vi "Live imaging-Generate images.vi"(4 "Left Channel":enum16{"Red Channel", "Green Channel"}(ring), 6 "Right Channel":enum16{"Red Channel", "Green Channel"}(ring), 10 "Images array":T1[](array[typedef]), 11 "Waveforms":waveform(dbl)[](array[waveform])) -> (0 "error out":errorcluster, 1 "Left image":T1, 3 "Right Image":T1)   [LabVIEW 2020]
uses:
  <vilib>/vision/Image Controls.llb/IMAQ Image.ctl
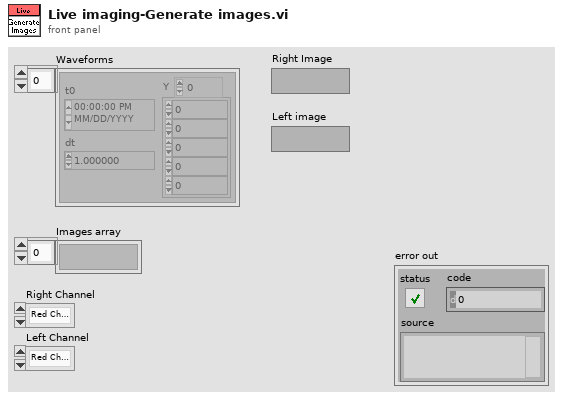
[diagram p1: front panel]
types:
  T1 = typedef "IMAQ Image.ctl" = refnum<image>
  T2 = typedef "AOL_Globals.ctl" = cluster{"Imaging Protocol":T3, "Number of POI":u16, "Number of Miniscans":u16, "Number of Trials":u16, "Number of Cycles ":u64, "# Averaged Frames":u16, "Laser power (%)":u8, "Pockels (V)":dbl, "Acquisition Length (sec)":dbl, "Fill time (us)":dbl, "POI Dwell time (us)":dbl, "Miniscan Dwell time per pixel (us)":dbl, "PMT 1":dbl, "PMT 2":dbl, "Back Apperture (mA)":dbl, "Frame Size":T4, "Center Frequency":dbl, "Field of View (norm)":dbl, "DwellTime (us)":dbl, "Wavelength (nm)":dbl, "Zoom":dbl, "AOL Z":dbl, "AOL Mode":T5, "GridXY":dbl, "GridZ":dbl, "TriggerPeriod (sec)":dbl, "Number of Pixels in Miniscan":u16, "Experiment folder path":path, "X centre":dbl, "Y centre":dbl, "Angle (degrees)":dbl, "Plane Mode":T6, "Threshold":u16[], "Regenerate Chirps":bool, "Rectangle ROI length (pixels)":u16, "Rectangle ROI height (pixels)":u16, "AOD fill":u16, "StartupDelay":i32, "Samples Wait after Trigger":u16, "Slip Cycle":u32, "Add Cycle":bool, "Functional Mode":T7, "Z Start":dbl, "Z Stop":dbl, "# Planes":i32, "Total Pixels":i32, "Variable Miniscan Pixels":u16[], "Use Variable Length":bool, "Use Variable Resolution":bool, "Laser power (%) at Z Start":u8, "Laser power (%) at Z Stop":u8, "Ref Z Step":i8, "Ref Dwell Time (us)":dbl, "Field of View (um)":dbl}
  T3 = typedef "Imaging Protocols enum.ctl" = enum16{"AOL Z-Stack", "Motor Z Stack", "Functional Acquisition", "Single Plane Acquisition", "Volume Acquisition", "Live Imaging", "Live Plane Imaging", "Live Volume Imaging"}
  T4 = typedef "Frame Size.ctl" = u16
  T5 = typedef "AOL modes.ctl" = enum16{"Raster", "Structural", "Pointing", "Mini Scan", "Alignment"}
  T6 = typedef "Plane Mode.ctl" = u16
  T7 = typedef "Functional Mode.ctl" = enum16{"Point", "Line", "Patch", "Plane", "Volume"}
  T8 = typedef "Live imaging queue element.ctl" = cluster{"Red channel":T1, "Green channel":T1, "Ref Red channel":T1, "Ref Green channel":T1, "Mov cor":bool}
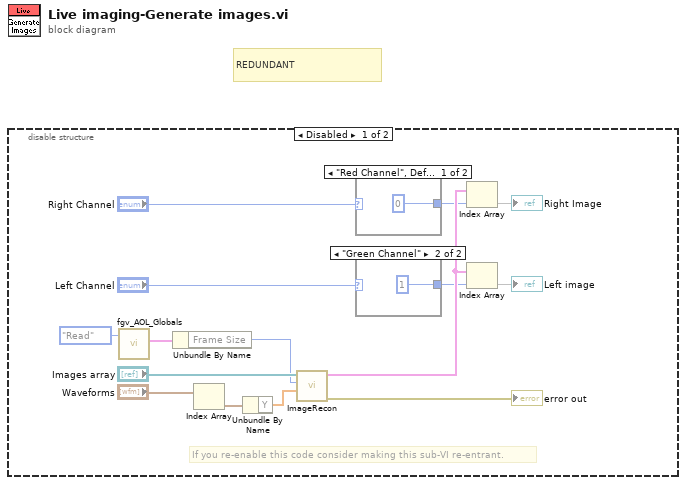
[diagram p0: block diagram]
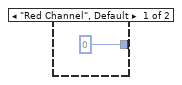
[diagram p2: hidden frame]
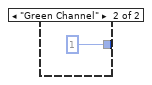
[diagram p3: hidden frame]
diagram:
  # "REDUNDANT"
  n1 = disable-structure shown="Disabled" {
    frame Disabled {
      # "If you re-enable this code consider making this sub-VI re-entrant."
      n2 = call "fgv_AOL_Globals.vi"("Function"=enum16{"Intialize", "Write", "Read", "Clear"}."Read") -> ("AOL_Globals"=w13:T2)  [unwired: 9 in, 1 out]
      n3 = Unbundle By Name(w13) -> ("Frame Size"=w4:T4)
      n4 = Index Array(array="Waveforms") -> (element=w3:waveform(dbl))  [unwired: 1 in]
      n5 = Unbundle By Name ("Get Waveform Components")(w3) -> ("Y"=w1:dbl[])
      n6 = call "ImageRecon.vi"("Data"=w1, "Frame Size"=w4, "Image Array (in)"="Images array") -> ("Error Out"=→"error out":errorcluster, "Image Array(out)"=w15:T8)  [unwired: 5 in, 2 out]
      n7 = case shown="\"Red Channel\", Default" "Right Channel" {
        tunnel: [0 ("index") 1 ("index")] -> w7
        frame "Red Channel", Default {
        }
        frame "Green Channel" {
        }
      }
      n8 = case shown="\"Green Channel\"" "Left Channel" {
        tunnel: [0 ("index") 1 ("index")] -> w8
        frame "Red Channel", Default {
        }
        frame "Green Channel" {
        }
      }
      n9 = Index Array(array=w15, index=w7) -> (element=→"Right Image")
      n10 = Index Array(array=w15, index=w8) -> (element=→"Left image")
    }
    frame Enabled {
    }
  }
